vi "WPI_CounterClose.vi"(8 "error in (no error)":errorcluster, 10 "Close Dependencies":bool=TRUE, 11 "CounterDevRef":T1) -> (0 "error out":errorcluster)   [LabVIEW 2017]
doc: "Closes the reference to the counter you specify. Use this VI to close each counter reference that you open with the Open VI. If you do not stop a running counter with the Stop VI, closing the reference to the counter stops the counter.\n\nThis software is licensed. Open the labview\\readme\\WPI Robotics Library Open Source License.txt file for more information."
uses:
  <vilib>/Rock Robotics/WPI/Counter/WPI_CounterDevRef.ctl
  <vilib>/Rock Robotics/SystemInterfaces/Counter/FPGA_CounterCtrSystemIndex.ctl
  <vilib>/Rock Robotics/WPI/Counter/WPI_CounterCacheOp.ctl
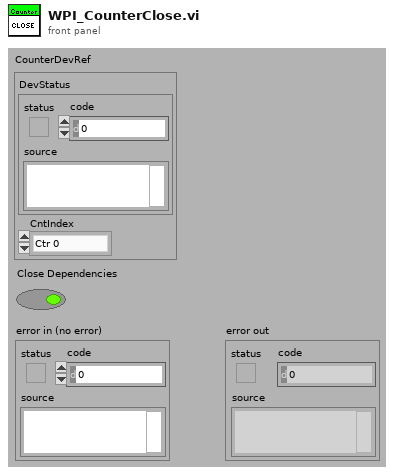
[diagram p1: front panel]
types:
  T1 = typedef "WPI_CounterDevRef.ctl" = cluster{"DevStatus":errorcluster, "CntIndex":T2}
  T2 = typedef "FPGA_CounterCtrSystemIndex.ctl" = enum8{"Ctr 0", "Ctr 1", "Ctr 2", "Ctr 3", "Ctr 4", "Ctr 5", "Ctr 6", "Ctr 7", "Invalid"}
  T3 = typedef "WPI_CounterCacheOp.ctl" = enum16{"Acquire", "Release"}
  T4 = typedef "FPGA_CounterEncoderSourceConvertionLVSourceType.ctl" = cluster{"DevStatus":errorcluster, "AnalogTriggerMode?":bool, "DigitalMode":cluster{"DIO Channel":T5}, "AnalogTriggerMode":cluster{"AnalogTriggerIndex":T6, "OutputType":T7}}
  T5 = typedef "FPGA_DIODigitalSourceChannel.ctl" = enum8{"DIO 0", "DIO 1", "DIO 2", "DIO 3", "DIO 4", "DIO 5", "DIO 6", "DIO 7", "DIO 8", "DIO 9", "DIO MXP 0", "DIO MXP 1", "DIO MXP 2", "DIO MXP 3", "DIO MXP 4", "DIO MXP 5", "DIO MXP 6", "DIO MXP 7", "DIO MXP 8", "DIO MXP 9", "DIO MXP 10", "DIO MXP 11", "DIO MXP 12", "DIO MXP 13", "DIO MXP 14", "DIO MXP 15", "Disabled"}
  T6 = typedef "FPGA_AnalogTriggerIndex.ctl" = enum8{"Trig 0", "Trig 1", "Trig 2", "Trig 3", "Trig 4", "Trig 5", "Trig 6", "Trig 7", "Invalid"}
  T7 = typedef "FPGA_AnalogTriggerOutType.ctl" = enum16{"InWindow", "TriggerState", "Rising", "Falling"}
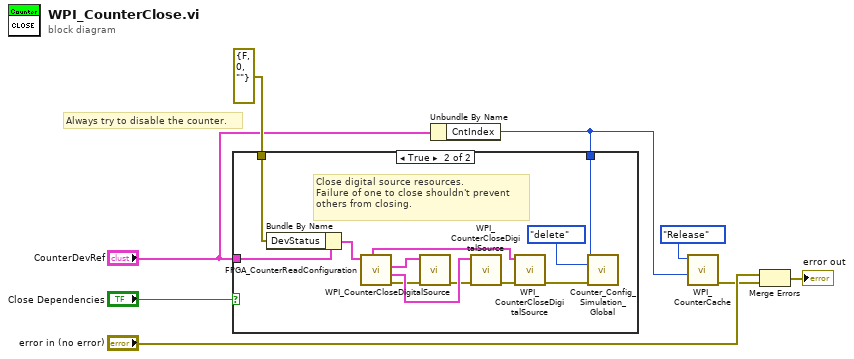
[diagram p0: block diagram]
diagram:
  # "Always try to disable the counter."
  n1 = Unbundle By Name("CounterDevRef") -> ("CntIndex"=w1:T2)
  n2 = case shown="True" "Close Dependencies" {
    tunnel: "CounterDevRef" -> [_ w16]
    tunnel: errorcluster {"status"=FALSE, "code"=0, "source"=""} ("DevStatus") -> [_ w14]
    tunnel: w1 -> [_ w10]
    frame False {
    }
    frame True {
      # "Close digital source resources.\nFailure of one to close shouldn't prevent\nothers from closing."
      n3 = Bundle By Name(cluster=w16, "DevStatus"=w14) -> (w15:T1)
      n4 = call <vilib>:"FPGA_CounterReadConfiguration.vi"("Ctr Ref in"=w15) -> ("error out"=w17:errorcluster, "DownSource"=w19:T4, "UpSource"=w20:T4, "Index Source"=w18:T4)  [unwired: 1 in, 6 out]
      n5 = call <vilib>:"WPI_CounterCloseDigitalSource.vi"("error in"=w17, "UpSource"=w20) -> ("error out"=w13:errorcluster)  [unwired: 5 out]
      n6 = call <vilib>:"WPI_CounterCloseDigitalSource.vi"("error in"=w13, "UpSource"=w19) -> ("error out"=w12:errorcluster)  [unwired: 5 out]
      n7 = call <vilib>:"WPI_CounterCloseDigitalSource.vi"("error in"=w12, "UpSource"=w18) -> ("error out"=w11:errorcluster)  [unwired: 5 out]
      n8 = call <vilib>:"Counter_Config_Simulation_Global.vi"("CntIndex"=w10, "menu"=enum16{"set", "get", "delete"}."delete", "error in (no error)"=w11) -> ()  [unwired: 11 in, 2 out]
    }
  }
  n9 = call <vilib>:"WPI_CounterCache.vi"("CntIndexToRelease"=w1, "Operation"=WPI_CounterCacheOp."Release") -> ("error out"=w4:errorcluster)  [unwired: 2 in, 7 out]
  n10 = Merge Errors("error in (no error)", w4) -> (→"error out":errorcluster)
